vi "Trigger Setting.vi"(7 "Trigger Resource (F:Internal)":bool, 8 "error in (no error)":errorcluster, 9 "Delay Aperture (0.500%)":dbl=0.5 min=0.5 max=100.0 format="%.4f", 10 "Delay Time (0.0 ms)":dbl min=0.0 max=3600000.0 format="%.3f", 11 "VISA resource name":refnum<visa-resource-name>) -> (0 "error out":errorcluster, 3 "VISA resource name out":refnum<visa-resource-name>)   [LabVIEW 2017, in "Agilent 4194.lvlib"]
doc: "This function sets the trigger resource, delay time, delay aperture."
uses:
  Agilent 4194.lvlib
panel:
  # "Ext/Manual"
  # "Internal"
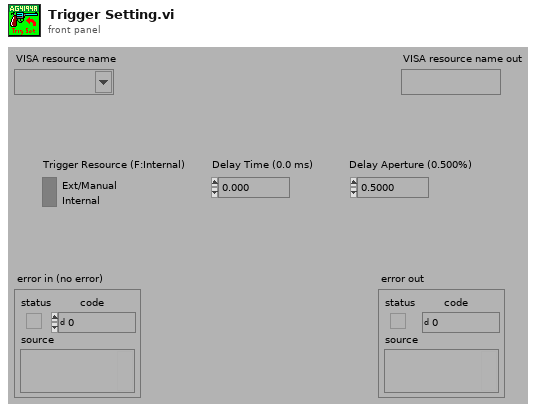
[diagram p1: front panel]
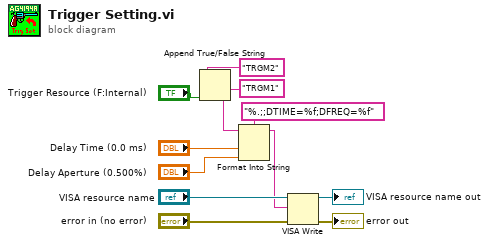
[diagram p0: block diagram]
diagram:
  n1 = Append True/False String(1:"Trigger Resource (F:Internal)", 2:"TRGM1", 3:"TRGM2") -> (0:w2:string)  [unwired: 1 in]
  n2 = Format Into String(format string="%.;;DTIME=%f;DFREQ=%f", initial string=w2, "Delay Time (0.0 ms)", "Delay Aperture (0.500%)") -> (resulting string=w1:string)  [unwired: 1 in, 1 out]
  n3 = VISA Write(VISA resource name="VISA resource name", write buffer=w1, error in (no error)="error in (no error)") -> (VISA resource name out=→"VISA resource name out":refnum<visa-resource-name>, error out=→"error out":errorcluster)  [unwired: 1 out]
